vi "read_tags_c-drum.vi"(8 "error in":errorcluster, 11 "Handle In":i32) -> (0 "error out":errorcluster, 2 "Read Data":T2 {"Drum Counter [counts]" format="%#_f"; "Flow Meter Volume [counts]" format="%#_f"; "Drum Position [counts]" format="%#_f"; "Drum Period [s]" format="%#_f"}, 3 "Handle Out":i32)   [LabVIEW 2025, in "LabJackEKG.lvlib"]
uses:
  LabJackEKG.lvlib
  Typedefs/ConnectionInfo.ctl
  Typedefs/ReadData.ctl
  Typedefs/AcqusitionConfig.ctl
  <vilib>/Platform/TimedLoop/XDataNode/timing_clust.ctl
  <vilib>/Platform/TimedLoop/XDataNode/nitl_modes.ctl
  <vilib>/Platform/TimedLoop/XDataNode/wakeup.ctl
  <vilib>/platform/TimedLoop/XDataNode/XDataNode.xnode
  <vilib>/Platform/TimedLoop/XDataNode/XDNodeRunTimeDep.lvlib
panel:
  in  "Acqusition Settings":T1 {"TC 2 Offset" format="%#_f"; "TC 2 Scale" format="%#_f"; "TC 1 Offset" format="%#_f"; "TC 1 Scale" format="%#_f"}
  in  "IPAddress":string="LJM_idANY"
  out "Connection Info":T3
  in  "Initialize":bool
  out "Response [ms]":dbl format="%.1f"
  in  "Period [ms]":i32=500 min=1 max=60000
  in  "Read Continuous":bool
  # "Driver Testing"
  # "note: To establish the direction, compare position in two consecutive reads. If a measured period is longer than the measurement period, the result might be zero."
  # "LabJack V0.10\nRead Drum/Flow Meter / TC"
  # "09.05.2025"
  # "Blaz Kelbl"
  # "Newtons4th V0.10\nRead"
  # "05.05.2025"
  # "Blaz Kelbl"
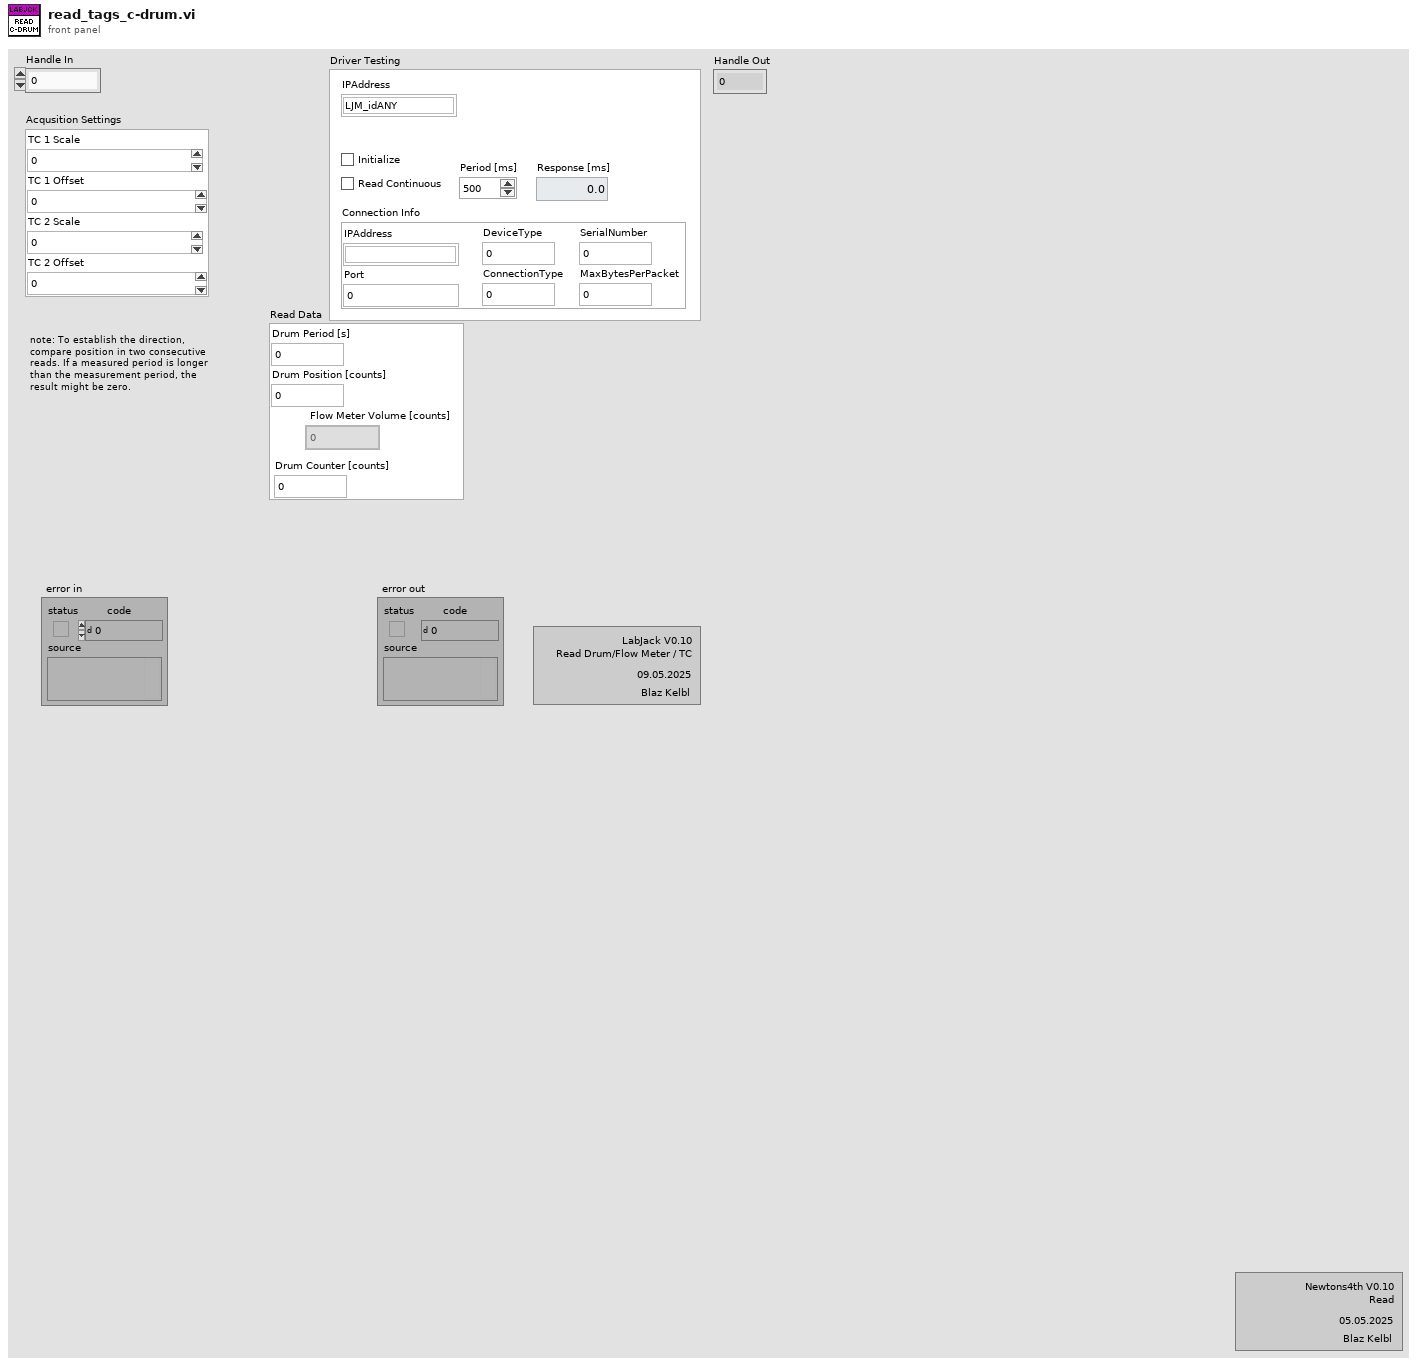
[diagram p1: front panel]
types:
  T1 = typedef "LabJackEKG.lvlib/AcqusitionConfig.ctl" = cluster{"TC 1 Scale":dbl, "TC 1 Offset":dbl, "TC 2 Scale":dbl, "TC 2 Offset":dbl}
  T2 = typedef "LabJackEKG.lvlib/ReadData.ctl" = cluster{"Drum Period [s]":dbl, "Drum Position [counts]":dbl, "Flow Meter Volume [counts]":dbl[], "Drum Counter [counts]":dbl}
  T3 = typedef "LabJackEKG.lvlib/ConnectionInfo.ctl" = cluster{"IPAddress":string, "Port":i32, "DeviceType":i32, "ConnectionType":i32, "SerialNumber":i32, "MaxBytesPerPacket":i32}
  T4 = typedef "XDNodeRunTimeDep.lvlib/timing_clust.ctl" = cluster{"Expected End [f-1]":u64, "Actual End [f-1]":u64, "Finished Late? [f-1]":bool, "Expected End [i-1]":u64, "Actual End [i-1]":u64, "Finished Late? [i-1]":bool, "Expected Start [i]":u64, "Actual Start [i]":u64, "Expected Start [f]":u64, "Actual Start [f]":u64, "Source Name":string, "Structure Name":string, "Period":i64, "Deadline":i64, "Offset":i64, "Start":i64, "Priority":i32, "Timeout":i32, "Mode":T5, "Wakeup Reason":T6, "Error":errorcluster, "Source Type":string, "Secondary Source Type":string, "Global End Time":u64, "Global Start Time":u64, "Frame Duration":u64, "Iteration Duration":u64, "Assigned CPU":i32, "I/O Scan Engine Mode":u32}
  T5 = typedef "XDNodeRunTimeDep.lvlib/nitl_modes.ctl" = enum32{"No Change", "Process missed periods, maintain original phase", "Discard missed periods, maintain original phase", "Process missed periods, ignore original phase", "Discard missed periods, ignore original phase"}
  T6 = typedef "XDNodeRunTimeDep.lvlib/wakeup.ctl" = enum32{"Normal", "Aborted", "Asynchronous wakeup", "Timing source error", "Timed loop error", "Timeout"}
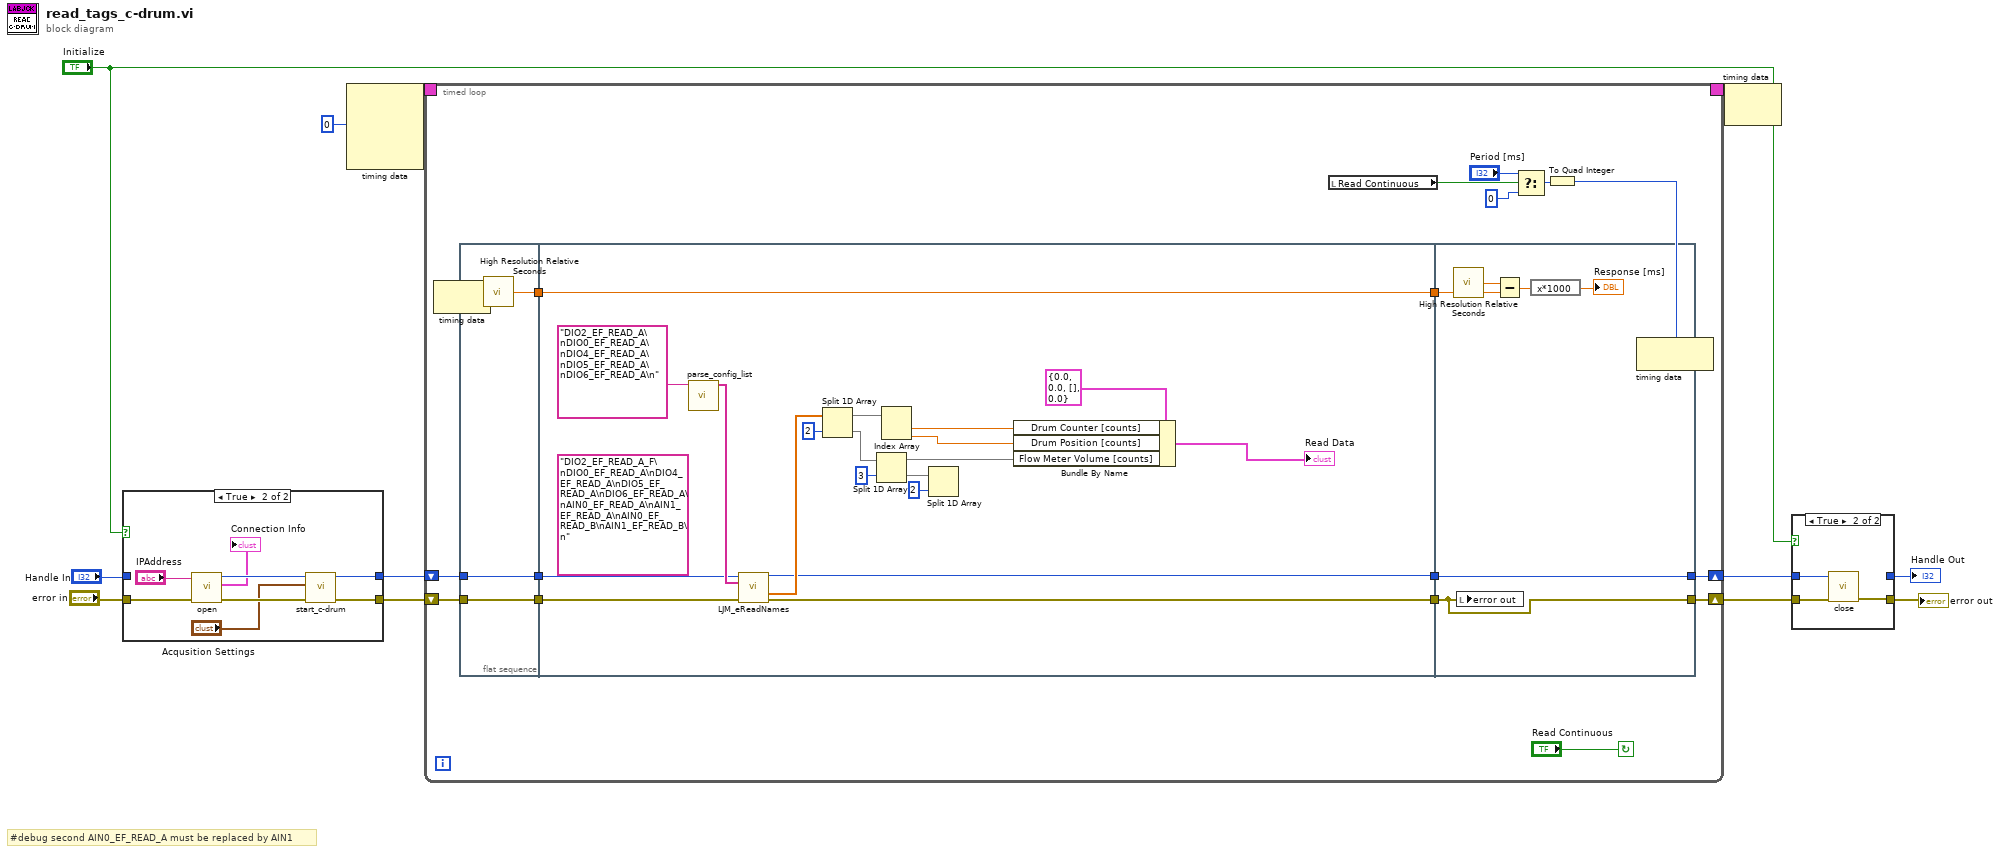
[diagram p0: block diagram]
diagram:
  # "#debug second AIN0_EF_READ_A must be replaced by AIN1"
  n1 = case shown="True" "Initialize" {
    tunnel: "error in" -> [w13 w22]
    tunnel: [w13 w17] -> w8
    tunnel: [w14 w18] -> w7
    tunnel: "Handle In" -> [w14 _]
    frame False {
    }
    frame True {
      n2 = call "open.vi"("error in"=w22, "IP Address (LJM_idANY )"="IPAddress") -> ("error out"=w21:errorcluster, "Connection Info"=→"Connection Info":T3, "Handle"=w20:i32)  [unwired: 7 in]
      n3 = call "start_c-drum.vi"("error in (no error)"=w21, "AcqConfig"="Acqusition Settings", "Handle In"=w20) -> ("error out"=w17:errorcluster, "Handle Out"=w18:i32)  [unwired: 7 in]
    }
  }
  n4 = node-c288(i64 0 ("Period")) -> (w12:T4)  [unwired: 3 in]
  n5 = timed-loop {
    timing: w12 -> [_]
    timing-out: [_] -> w11
    shift-right: [w29] -> w5
    shift-left: w8 -> [w32]
    shift-right: [w33] -> w6
    shift-left: w7 -> [w34]
    stop <- "Read Continuous" continue-if-true
    n6 = node-c288() -> ()  [unwired: 1 in, 1 out]
    n7 = flat-sequence {
      tunnel: w32 -> [w40]
      tunnel: w34 -> [w41]
      tunnel: [w41] -> w28
      tunnel: [w40] -> w27
      tunnel: [w39] -> w25
      tunnel: [w42] -> w31
      tunnel: [w56] -> w30
      tunnel: w28 -> [w57]
      tunnel: w27 -> [w55]
      tunnel: [w60] -> w26
      tunnel: w25 -> [w60]
      tunnel: [w65] -> w29
      tunnel: [w66] -> w33
      tunnel: w31 -> [w66]
      tunnel: w30 -> [w65]
      tunnel: w26 -> [w62]
      frame #0 {
        n8 = call <vilib>:"High Resolution Relative Seconds.vi"() -> ("relative seconds"=w39:dbl)
      }
      frame #1 {
        (unwired) "DIO2_EF_READ_A_F\nDIO0_EF_READ_A\nDIO4_EF_READ_A\nDIO5_EF_READ_A\nDIO6_EF_READ_A\nAIN0_EF_READ_A\nAIN1_EF_READ_A\nAIN0_EF_READ_B\nAIN1_EF_READ_B\n" ("String")
        n9 = call "parse_config_list.vi"("String"="DIO2_EF_READ_A\nDIO0_EF_READ_A\nDIO4_EF_READ_A\nDIO5_EF_READ_A\nDIO6_EF_READ_A\n") -> ("Names"=w58:string[])  [unwired: 9 in, 1 out]
        n10 = call <vilib>:"LJM_eReadNames.vi"("Handle In"=w57, "aNames"=w58, "error in"=w55) -> ("Handle Out"=w42:i32, "aValuesOut"=w51:dbl[], "error out"=w56:errorcluster)  [unwired: 9 in, 1 out]
        n11 = Split 1D Array(array=w51, index=2) -> (first subarray=w50:dbl[], second subarray=w47:dbl[])
        n12 = Split 1D Array(array=w47, index=3) -> (first subarray=w46:dbl[], second subarray=w44:dbl[])
        n13 = Index Array(array=w50) -> (element #1=w53:dbl, element #2=w52:dbl)  [unwired: 2 in]
        n14 = Split 1D Array(array=w44, index=2) -> ()  [unwired: 2 out]
        n15 = Bundle By Name(cluster=T2 {"Drum Period [s]"=0.0, "Drum Position [counts]"=0.0, "Flow Meter Volume [counts]"=[], "Drum Counter [counts]"=0.0} ("Read Data"), "Drum Counter [counts]"=w53, "Drum Position [counts]"=w52, "Flow Meter Volume [counts]"=w46) -> (→"Read Data":T2)
      }
      frame #2 {
        n16 = call <vilib>:"High Resolution Relative Seconds.vi"() -> ("relative seconds"=w64:dbl)
        n17 = local write "error out"(w65) -> ()
        n18 = Subtract(x=w64, y=w62) -> (x-y=w63:dbl)
        n19 = expression code="x*1000"(w63) -> (→"Response [ms]":dbl)
      }
    }
    n20 = local read "Read Continuous"() -> (w38:bool)
    n21 = Select(t="Period [ms]", s=w38, f=0) -> (s? t:f=w36:i32)
    n22 = To Quad Integer(1:w36) -> (0:w35:i64)
    n23 = node-c288(w35) -> ()  [unwired: 1 out]
  }
  n24 = node-c288(w11) -> ()  [unwired: 1 out]
  n25 = case shown="True" "Initialize" {
    tunnel: w6 -> [w72 w73]
    tunnel: w5 -> [w71 w75]
    tunnel: [w72 _] -> w1
    tunnel: [w71 w74] -> w4
    frame False {
    }
    frame True {
      n26 = call "close.vi"("error in"=w75, "Handle"=w73) -> ("error out"=w74:errorcluster)  [unwired: 9 in]
    }
  }
  "error out" <- w4
  "Handle Out" <- w1
